vi "External Transition.vi"(8 "error in (no error)":errorcluster, 10 "Target":refnum<class "State Machine.lvclass">, 11 "State Machine in":refnum<class "State Machine.lvclass">) -> (0 "error out":errorcluster, 3 "State Machine out":refnum<class "State Machine.lvclass">)   [LabVIEW 2024]
uses:
  State Machine.lvclass
  State Machine.lvclass/State Machine.ctl
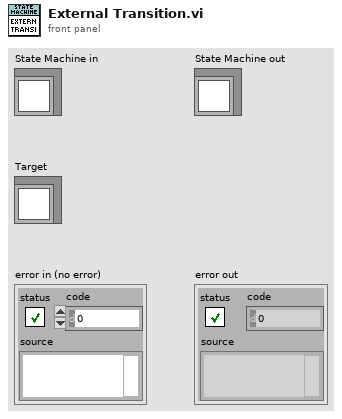
[diagram p1: front panel]
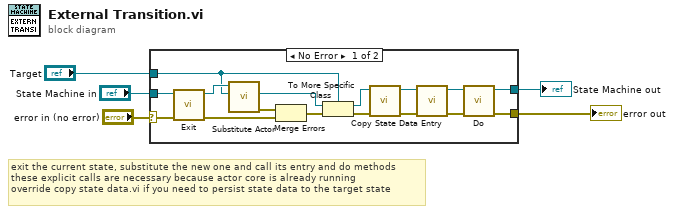
[diagram p0: block diagram]
diagram:
  # "exit the current state, substitute the new one and call its entry and do methods\nthese explicit calls are necessary because actor core is already running\noverride copy state data.vi if you need to persist state data to the target state"
  n1 = case shown="No Error" "error in (no error)" {
    selector: "error in (no error)" -> [w15 w23]
    tunnel: [w13 w23] -> w4
    tunnel: [w19 w22] -> w2
    tunnel: "State Machine in" -> [w21 w22]
    tunnel: "Target" -> [w16 _]
    frame No Error {
      n2 = call-dynamic "Exit.vi"("error in (no error)"=w15, "State Machine in"=w21) -> ("error out"=w11:errorcluster, "State Machine out"=w18:refnum<class "State Machine.lvclass">)  [unwired: 8 in]
      n3 = call-dynamic "Substitute Actor.vi"("Substitute Actor in"=w16, "Current Actor"=w18) -> ("error out"=w12:errorcluster, "Substitute Actor out"=w17:refnum<class "Actor.lvclass">)  [unwired: 8 in]
      n4 = Merge Errors(w12, w11) -> (w10:errorcluster)
      n5 = To More Specific Class(target class=w16, reference=w17, error in=w10) -> (specific class reference=w9:refnum<class "State Machine.lvclass">, error out=w7:errorcluster)
      n6 = call-dynamic "Copy State Data.vi"("error in (no error)"=w7, "State Machine in"=w9) -> ("error out"=w6:errorcluster, "State Machine out"=w8:refnum<class "State Machine.lvclass">)  [unwired: 8 in]
      n7 = call-dynamic "Entry.vi"("error in (no error)"=w6, "State Machine in"=w8) -> ("error out"=w14:errorcluster, "State Machine out"=w20:refnum<class "State Machine.lvclass">)  [unwired: 8 in]
      n8 = call-dynamic "Do.vi"("error in (no error)"=w14, "State Machine in"=w20) -> ("error out"=w13:errorcluster, "State Machine out"=w19:refnum<class "State Machine.lvclass">)  [unwired: 8 in]
    }
    frame Error {
    }
  }
  "error out" <- w4
  "State Machine out" <- w2
